vi "7 segment.vi"() -> ()   [LabVIEW 2018]
panel:
  out "7 2":bool
  out "6 2":bool
  out "5 2":bool
  out "4 2":bool
  out "3 2":bool
  out "2 2":bool
  out "1 2":bool
  out "7":bool
  out "6":bool
  out "5":bool
  out "4":bool
  out "3":bool
  out "2":bool
  out "1":bool
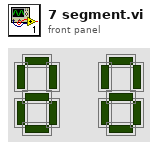
[diagram p1: front panel]
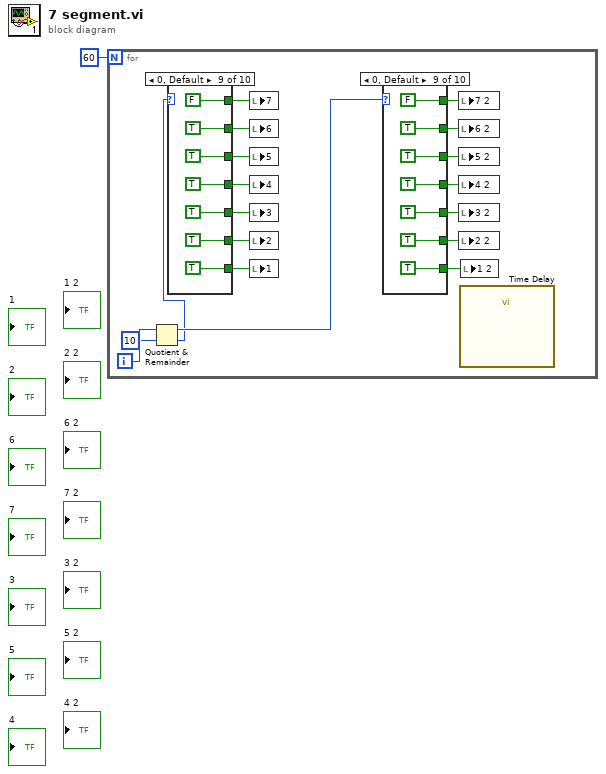
[diagram p0: block diagram]
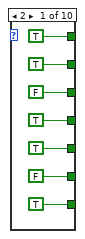
[diagram p2: hidden frame]
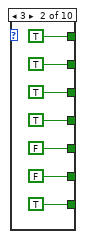
[diagram p3: hidden frame]
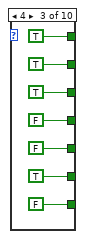
[diagram p4: hidden frame]
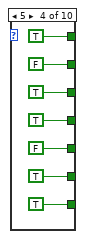
[diagram p5: hidden frame]
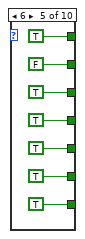
[diagram p6: hidden frame]
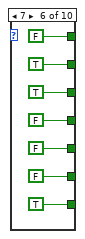
[diagram p7: hidden frame]
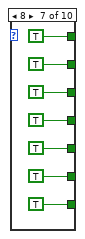
[diagram p8: hidden frame]
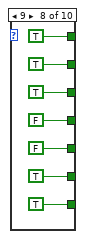
[diagram p9: hidden frame]
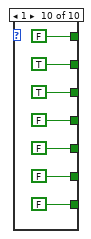
[diagram p10: hidden frame]
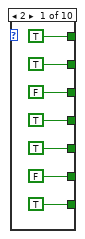
[diagram p11: hidden frame]
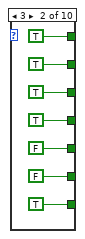
[diagram p12: hidden frame]
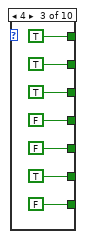
[diagram p13: hidden frame]
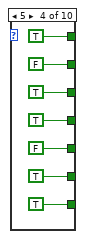
[diagram p14: hidden frame]
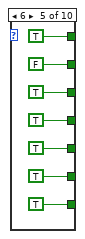
[diagram p15: hidden frame]
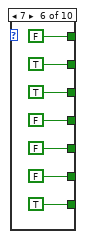
[diagram p16: hidden frame]
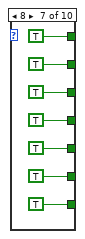
[diagram p17: hidden frame]
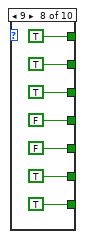
[diagram p18: hidden frame]
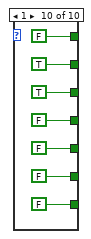
[diagram p19: hidden frame]
diagram:
  n1 = for {
    N: 60 -> [_]
    i -> [w5]
    n2 = Quotient & Remainder(x=w5, y=10) -> (x-y*floor(x/y)=w3:i32, floor(x/y)=w2:i32)
    n3 = case shown="0, Default" w2 {
      tunnel: [TRUE TRUE FALSE TRUE TRUE TRUE TRUE TRUE TRUE FALSE] -> w19
      tunnel: [FALSE FALSE TRUE TRUE TRUE FALSE TRUE TRUE TRUE FALSE] -> w18
      tunnel: [TRUE FALSE FALSE FALSE TRUE FALSE TRUE FALSE TRUE FALSE] -> w17
      tunnel: [TRUE TRUE FALSE TRUE TRUE FALSE TRUE FALSE TRUE FALSE] -> w16
      tunnel: [FALSE TRUE TRUE TRUE TRUE TRUE TRUE TRUE TRUE TRUE] -> w15
      tunnel: [TRUE TRUE TRUE FALSE FALSE TRUE TRUE TRUE TRUE TRUE] -> w14
      tunnel: [TRUE TRUE TRUE TRUE TRUE FALSE TRUE TRUE FALSE FALSE] -> w13
      frame 2 {
      }
      frame 3 {
      }
      frame 4 {
      }
      frame 5 {
      }
      frame 6 {
      }
      frame 7 {
      }
      frame 8 {
      }
      frame 9 {
      }
      frame 0, Default {
      }
      frame 1 {
      }
    }
    n4 = local write "7"(w13) -> ()
    n5 = local write "6"(w14) -> ()
    n6 = local write "5"(w15) -> ()
    n7 = local write "4"(w16) -> ()
    n8 = local write "3"(w17) -> ()
    n9 = local write "2"(w18) -> ()
    n10 = local write "1"(w19) -> ()
    n11 = case shown="0, Default" w3 {
      tunnel: [TRUE TRUE FALSE TRUE TRUE TRUE TRUE TRUE TRUE FALSE] -> w12
      tunnel: [FALSE FALSE TRUE TRUE TRUE FALSE TRUE TRUE TRUE FALSE] -> w11
      tunnel: [TRUE FALSE FALSE FALSE TRUE FALSE TRUE FALSE TRUE FALSE] -> w10
      tunnel: [TRUE TRUE FALSE TRUE TRUE FALSE TRUE FALSE TRUE FALSE] -> w9
      tunnel: [FALSE TRUE TRUE TRUE TRUE TRUE TRUE TRUE TRUE TRUE] -> w8
      tunnel: [TRUE TRUE TRUE FALSE FALSE TRUE TRUE TRUE TRUE TRUE] -> w7
      tunnel: [TRUE TRUE TRUE TRUE TRUE FALSE TRUE TRUE FALSE FALSE] -> w6
      frame 2 {
      }
      frame 3 {
      }
      frame 4 {
      }
      frame 5 {
      }
      frame 6 {
      }
      frame 7 {
      }
      frame 8 {
      }
      frame 9 {
      }
      frame 0, Default {
      }
      frame 1 {
      }
    }
    n12 = local write "7 2"(w6) -> ()
    n13 = local write "6 2"(w7) -> ()
    n14 = local write "5 2"(w8) -> ()
    n15 = local write "4 2"(w9) -> ()
    n16 = local write "3 2"(w10) -> ()
    n17 = local write "2 2"(w11) -> ()
    n18 = call "Time Delay"() -> ()  [unwired: 11 in, 1 out]
    n19 = local write "1 2"(w12) -> ()
  }
